vi "qCST.vi"(0 "System no.":i32=1 min=1 max=4 step=1, 2 "Axes to query":string[](array[string]), 3 "All Axes?":bool, 4 "Axis Identifier?":bool=TRUE, 5 "error in":errorcluster) -> (14 "Stage names":string[](array[string]), 19 "error out":errorcluster)   [LabVIEW 2026]
doc: "Returns the name of the connected stage for queried axes.\n\nC-702, C-843, C-843.PM, C-844, C-848, C-880, C-887, F-206, M-8X0: If All axes? = TRUE, then Axis identifier? must be TRUE\n\nC-413, C-865, C-866, C-867, C-877, C-884, C-885, C-891, E-135, E-709, E-710, E-712, E-725, E-727, E-753, E-754, E-755, E-761, E-861, E-871, E-873, E-874, Hydra, Mercury, Mercury_GCS: If All axes? = TRUE, then Axis identifier? can be FALSE\n\nC-887, F-206, M-8X0: Check HLP?/HELP answer to find out if CST? is supported\n\nPollux: If All axes? = TRUE, then Axis identifier? can be FALSE. See HydraPollux_GCS_DLL Manual for specialities of the Pollux controller family regarding stage name settings."
panel:
  # "Returns the name of the connected stage for queried axes."
  # "If all axes: use"
  # "Query"
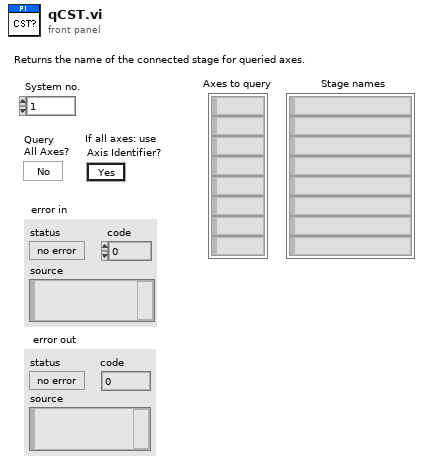
[diagram p1: front panel]
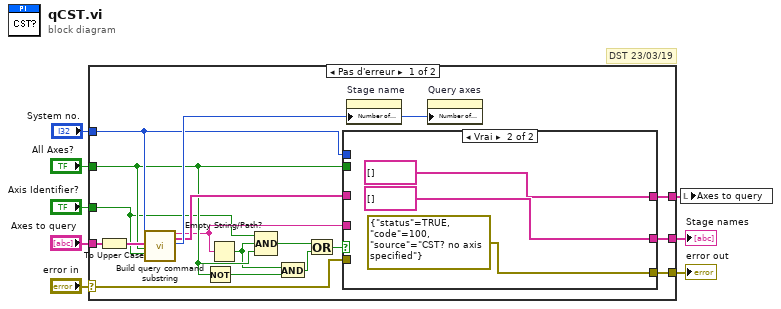
[diagram p0: block diagram]
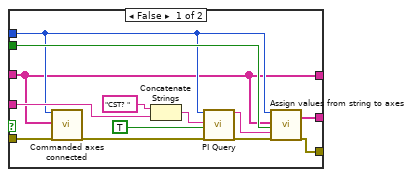
[diagram p2: hidden frame]
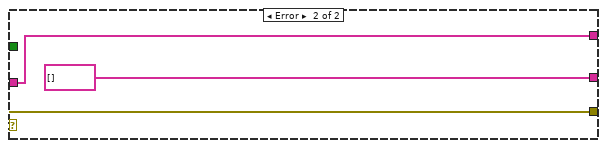
[diagram p3: hidden frame]
diagram:
  # "DST 23/03/19"
  n1 = case shown="Pas d'erreur" "error in" {
    selector: "error in" -> [w10 w43]
    tunnel: "Axes to query" -> [w25 w42]
    tunnel: [w24 w43] -> w7
    tunnel: "System no." -> [w21 _]
    tunnel: "Axis Identifier?" -> [w11 _]
    tunnel: "All Axes?" -> [w17 _]
    tunnel: [w15 string[] [] ("Strings")] -> w3
    tunnel: [w9 w42] -> w1
    frame No Error {
      n2 = To Upper Case(1:w25) -> (0:w23:string[])
      n3 = call "Build query command substring.vi"("System no."=w21, "Axes to query in"=w23, "Query\nAll axes?"=w17, "For all axes: use\nAxis identifier?"=w11) -> ("Command substring"=w14:string, "Axes to query out"=w20:string[], "Number of rows"=w22:u32)  [unwired: 2 in, 11 out]
      n4 = Not(x=w17) -> (.not. x?=w19:bool)
      n5 = Empty String/Path?(string/path=w14) -> (empty?=w13:bool)
      n6 = Compound Arithmetic op=AND(w11, w13, w17) -> (w16:bool)
      n7 = And(x=w13, y=w19) -> (x .and. y?=w18:bool)
      n8 = Or(x=w16, y=w18) -> (x .or. y?=w12:bool)
      n9 = case shown="Vrai" w12 {
        tunnel: w10 -> [w35 _]
        tunnel: [w34 errorcluster {"status"=TRUE, "code"=100, "source"="CST? no axis specified"} ("error out")] -> w24
        tunnel: w21 -> [w27 _]
        tunnel: w20 -> [w26 _]
        tunnel: w17 -> [w33 _]
        tunnel: [w32 string[] [] ("Strings")] -> w15
        tunnel: w14 -> [w28 _]
        tunnel: [w26 string[] [] ("Axes to query out")] -> w9
        frame False {
          n10 = call "Commanded axes connected.vi"("System no."=w27, "Commanded axes"=w26, "error in"=w35) -> ("error out"=w31:errorcluster)  [unwired: 1 in, 15 out]
          n11 = Concatenate Strings("CST? ", w28) -> (w36:string)
          n12 = call "PI Query.vi"("System no."=w27, "String to send"=w36, "Attach termination char.?"=TRUE ("Attach Linefeed?"), "error in"=w31) -> ("String read"=w30:string, "error out"=w29:errorcluster)  [unwired: 3 in, 11 out]
          n13 = call "Assign values from string to axes.vi"("System no."=w27, "Queried axes"=w26, "All axes queried?"=w33, "Input String"=w30, "error in"=w29) -> ("Strings"=w32:string[], "error out"=w34:errorcluster)  [unwired: 4 in, 9 out]
        }
        frame True {
        }
      }
      n14 = property on="Stage name" class="Tabl (strict)"("Number of Rows"=w22) -> ()  [unwired: 2 in, 2 out]
      n15 = property on="Query axes" class="Tabl (strict)"("Number of Rows"=w22) -> ()  [unwired: 2 in, 2 out]
    }
    frame Error {
    }
  }
  "error out" <- w7
  "Stage names" <- w3
  n16 = local write "Axes to query"(w1) -> ()
